vi "Detect Controller.vi"(4 "Expose System Hardware Reference":bool caption="Expose System Hardware Reference (F)", 6 "Network Adapters":bool caption="Network Adapters (F)", 8 "error in":errorcluster, 11 "Device in":refnum<class "SysCfg Device.lvclass">) -> (0 "error out":errorcluster, 2 "Controller out":refnum<class "Controller.lvclass">, 3 "Device out":refnum<class "SysCfg Device.lvclass">)   [LabVIEW 2015, in "SMI.lvlib" / "Controller.lvclass"]
uses:
  Controller.lvclass
  SysCfg Device/SysCfg Device.lvclass
  SysCfg Device/SysCfg Device.lvclass/SysCfg Device.ctl
  Device/Device.lvclass/Device.ctl
  Controller.lvclass/Controller.ctl
  SysCfg Device/Read SysCfg Session.vi
  SysCfg Device/Write SysCfg Session.vi
  Device/Accessor Methods/Write Vendor Name.vi
  Device/Accessor Methods/Write Product Name.vi
  Device/Accessor Methods/Write Product ID.vi
  Device/Accessor Methods/Write Serial Number.vi
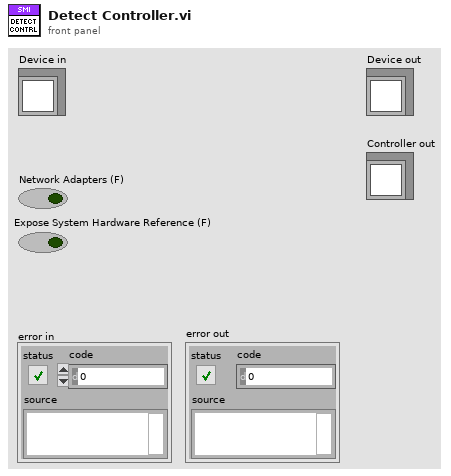
[diagram p1: front panel]
types:
  T1 = typedef "SMI.lvlib/Controller.lvclass/NetworkDevice.ctl" = cluster{"System Hardware Reference":refnum<k20>, "Vendor Name":string, "Product Name":string, "Product ID":u32, "Serial Number":string, "Device Information":T2, "Primary Network Adapter":T3, "Secondary Network Adapters":T3[]}
  T2 = typedef "SMI.lvlib/Controller.lvclass/DeviceInformation.ctl" = cluster{"Resource":string, "Device Class":string, "System Start Time":timestamp, "Current Time":timestamp, "Time Zone":string, "Firmware Revision":string, "Image Title":string, "Image Version":string, "System Status":string, "Credential type":enum16{"None/Unlocked", "FTP Password", "NIAuth Credentials"}, "User Added":bool}
  T3 = typedef "SMI.lvlib/Controller.lvclass/NetworkAdapterSettings.ctl" = cluster{"IP Address":string, "MAC Address":string, "IP Address Request Mode":u32, "SubnetMask":string, "Gateway":string, "DNS Server":string, "Adapter Mode":u32, "Adapter Type":u32}
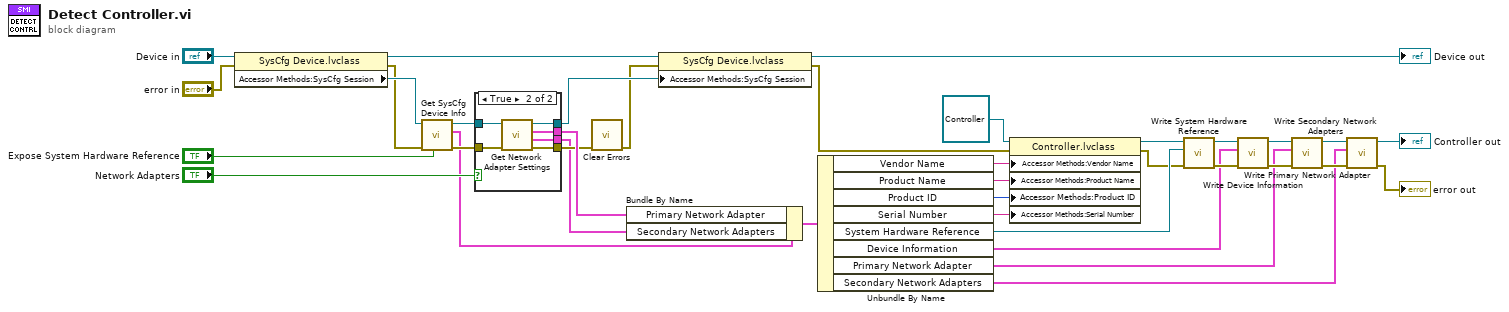
[diagram p0: block diagram]
diagram:
  n1 = property class="SysCfg Device.lvclass"(reference="Device in", error in="error in") -> (reference out=w26:refnum<class "SysCfg Device.lvclass">, error out=w27:errorcluster, "Accessor Methods:SysCfg Session"=w29:refnum<k21>)
  n2 = call "Get SysCfg Device Info.vi"("Expose System Hardware Reference"="Expose System Hardware Reference", "error in"=w27, "Refnum in"=w29) -> ("error out"=w35:errorcluster, "Network Device"=w32:T1, "Refnum out"=w36:refnum<k21>)  [unwired: 6 in]
  n3 = case shown="True" "Network Adapters" {
    tunnel: w36 -> [w39 w45]
    tunnel: w35 -> [w38 w44]
    tunnel: [_ w43] -> w34
    tunnel: [w39 w42] -> w25
    tunnel: [w38 w41] -> w33
    tunnel: [_ w40] -> w31
    frame False {
    }
    frame True {
      n4 = call "Get Network Adapter Settings.vi"("error in"=w44, "Refnum in"=w45) -> ("error out"=w41:errorcluster, "Secondary Network Adapters"=w40:T3[], "Primary Network Adapter"=w43:T3, "Refnum out"=w42:refnum<k21>)  [unwired: 6 in]
    }
  }
  n5 = call <vilib>:"Clear Errors.vi"("error in (no error)"=w33) -> ("error out"=w23:errorcluster)  [unwired: 5 in, 1 out]
  n6 = Bundle By Name(cluster=w32, "Primary Network Adapter"=w34, "Secondary Network Adapters"=w31) -> (w21:T1)
  n7 = property class="SysCfg Device.lvclass"(reference=w26, error in=w23, "Accessor Methods:SysCfg Session"=w25) -> (reference out=→"Device out":refnum<class "SysCfg Device.lvclass">, error out=w6:errorcluster)
  n8 = Unbundle By Name(w21) -> ("Vendor Name"=w4:string, "Product Name"=w3:string, "Product ID"=w2:u32, "Serial Number"=w1:string, "System Hardware Reference"=w12:refnum<k20>, "Device Information"=w11:T2, "Primary Network Adapter"=w10:T3, "Secondary Network Adapters"=w9:T3[])
  n9 = property class="Controller.lvclass"(reference=refnum<class "Controller.lvclass"> refnum ("SMI.lvlib:Controller.lvclass"), error in=w6, "Accessor Methods:Vendor Name"=w4, "Accessor Methods:Product Name"=w3, "Accessor Methods:Product ID"=w2, "Accessor Methods:Serial Number"=w1) -> (reference out=w7:refnum<class "Controller.lvclass">, error out=w5:errorcluster)
  n10 = call "Write System Hardware Reference.vi"("error in (no error)"=w5, "System Hardware Reference"=w12, "Controller in"=w7) -> ("error out"=w16:errorcluster, "Controller out"=w17:refnum<class "Controller.lvclass">)  [unwired: 7 in]
  n11 = call "Write Device Information.vi"("error in (no error)"=w16, "Device Information"=w11, "Controller in"=w17) -> ("error out"=w15:errorcluster, "Controller out"=w18:refnum<class "Controller.lvclass">)  [unwired: 7 in]
  n12 = call "Write Primary Network Adapter.vi"("error in (no error)"=w15, "Network Adapter Settings"=w10, "Controller in"=w18) -> ("error out"=w19:errorcluster, "Controller out"=w20:refnum<class "Controller.lvclass">)  [unwired: 7 in]
  n13 = call "Write Secondary Network Adapters.vi"("error in (no error)"=w19, "Secondary Network Adapters"=w9, "Controller in"=w20) -> ("error out"=→"error out":errorcluster, "Controller out"=→"Controller out":refnum<class "Controller.lvclass">)  [unwired: 7 in]
